vi "temperature.vi"(8 "error in (no error)":errorcluster) -> (0 "error out":errorcluster, 2 "Temperature (C)":dbl)   [LabVIEW 2013]
doc: "Random temperature generator centered at 20C with a Gaussian statistical distribution."
uses:
  <vilib>/Analysis/NI_AALBase.lvlib
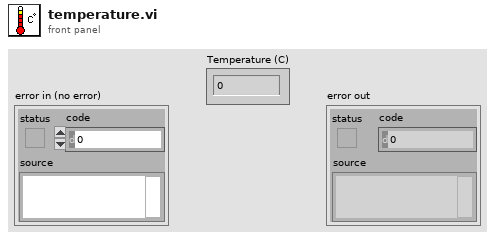
[diagram p1: front panel]
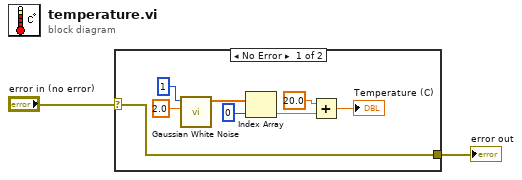
[diagram p0: block diagram]
diagram:
  n1 = case shown="No Error" "error in (no error)" {
    selector: "error in (no error)" -> [w3 w11]
    tunnel: [w3 w11] -> w1
    frame No Error {
      n2 = call <vilib>:"Gaussian White Noise.vi"("standard deviation"=2.0, "samples"=1) -> ("Gaussian noise pattern"=w8:dbl[])  [unwired: 8 in, 1 out]
      n3 = Index Array(array=w8, index=0) -> (element=w6:dbl)
      n4 = Add(x=20.0, y=w6) -> (x+y=→"Temperature (C)":dbl)
    }
    frame Error {
    }
  }
  "error out" <- w1
